vi "Get Next Service State.vi"(8 "error in (no error)":errorcluster) -> (0 "error out":errorcluster, 3 "Service States":T1)   [LabVIEW 2016, in "Assert API Components.lvlib" / "Assert Service.lvlib" / "Assert Service.lvclass"]
uses:
  Assert Service.lvclass
  Service States.ctl
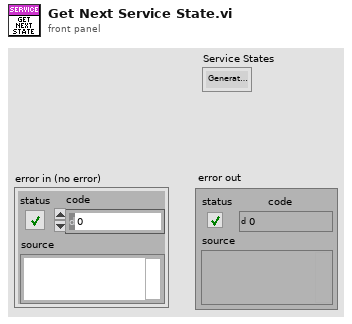
[diagram p1: front panel]
types:
  T1 = typedef "Service States.ctl" = enum16{"Generate Link", "Acquire Data"}
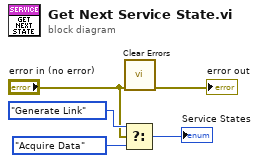
[diagram p0: block diagram]
diagram:
  n1 = Select(t=Service_States."Generate Link", s="error in (no error)", f=Service_States."Acquire Data") -> (s? t:f=→"Service States":T1)
  n2 = call <vilib>:"Clear Errors.vi"("error in (no error)"="error in (no error)") -> ("error out"=→"error out":errorcluster)  [unwired: 5 in, 1 out]
